vi "SVI_VoltageToDAC_IntegerString.vi"(1 "Voltage Limits":cluster{"Maximum":dbl, "Minimum":dbl}, 2 "Divisions (Precision)":i32=4096, 3 "Set Voltage":dbl) -> (0 "DAC Int String":string)   [LabVIEW 2014]
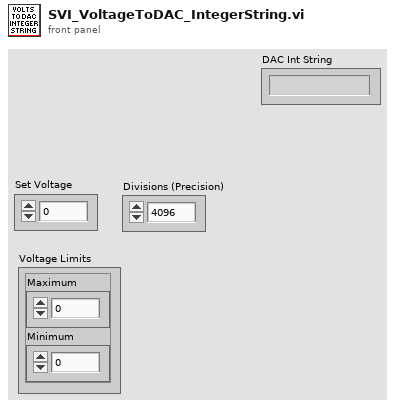
[diagram p1: front panel]
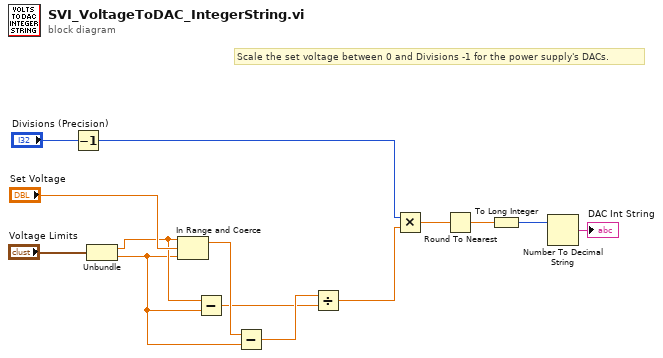
[diagram p0: block diagram]
diagram:
  # "Scale the set voltage between 0 and Divisions -1 for the power supply's DACs."
  n1 = Decrement(x="Divisions (Precision)") -> (x-1=w7:i32)
  n2 = Unbundle("Voltage Limits") -> ("Maximum"=w2:dbl, "Minimum"=w1:dbl)
  n3 = In Range and Coerce(upper limit=w2, x="Set Voltage", lower limit=w1) -> (coerced(x)=w12:dbl)  [unwired: 1 out]
  n4 = Subtract(x=w2, y=w1) -> (x-y=w10:dbl)
  n5 = Subtract(x=w12, y=w1) -> (x-y=w11:dbl)
  n6 = Divide(x=w11, y=w10) -> (x/y=w8:dbl)
  n7 = Multiply(x=w7, y=w8) -> (x*y=w6:dbl)
  n8 = Round To Nearest(number=w6) -> (nearest integer value=w5:dbl)
  n9 = To Long Integer(number=w5) -> (32bit integer=w4:i32)
  n10 = Number To Decimal String(number=w4) -> (decimal integer string=→"DAC Int String":string)  [unwired: 1 in]
